vi "bmi_calculator.vi"() -> ()   [LabVIEW 2020]
panel:
  out "BMI Calculation":dbl
  in  "Cases":T1(ring)
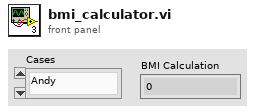
[diagram p1: front panel]
types:
  T1 = enum16{"Andy", "Belinda", "Christina", "David", "Eric"}
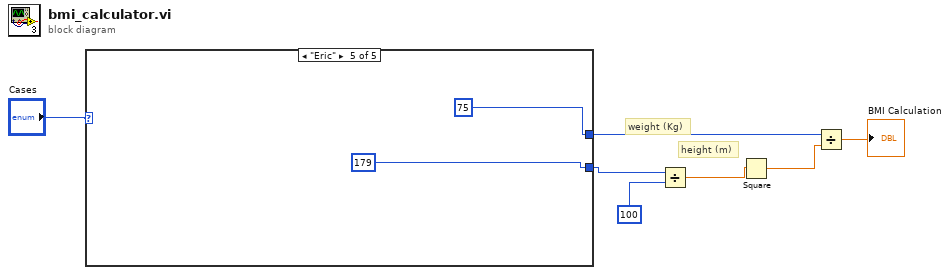
[diagram p0: block diagram]
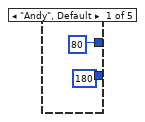
[diagram p2: hidden frame]
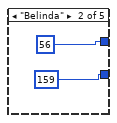
[diagram p3: hidden frame]
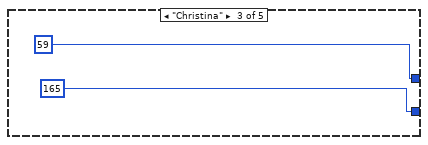
[diagram p4: hidden frame]
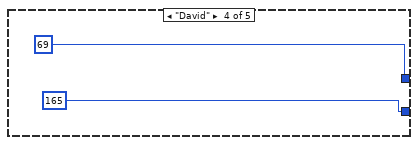
[diagram p5: hidden frame]
diagram:
  # "height (m)"
  # "weight (Kg)"
  n1 = case shown="\"Eric\"" "Cases" {
    tunnel: [180 159 165 165 179] -> w3
    tunnel: [80 56 59 69 75] -> w6
    frame "Andy", Default {
    }
    frame "Belinda" {
    }
    frame "Christina" {
    }
    frame "David" {
    }
    frame "Eric" {
    }
  }
  n2 = Divide(x=w3, y=100) -> (x/y=w1:dbl)
  n3 = Square(x=w1) -> (x^2=w5:dbl)
  n4 = Divide(x=w6, y=w5) -> (x/y=→"BMI Calculation":dbl)
